vi "SensorSerialReceiver.vi"(8 "Notifier Error In":errorcluster, 9 "Notifier":refnum<notifier>, 10 "Queue":refnum<queue>, 11 "COM Port":refnum<visa-resource-name>="COM6") -> (0 "Notifier Error Out":errorcluster, 3 "Done":bool=TRUE)   [LabVIEW 2013]
uses:
  <vilib>/Instr/_visa.llb/VISA Configure Serial Port (Instr).vi
panel:
  in  "baud rate":u32=115200
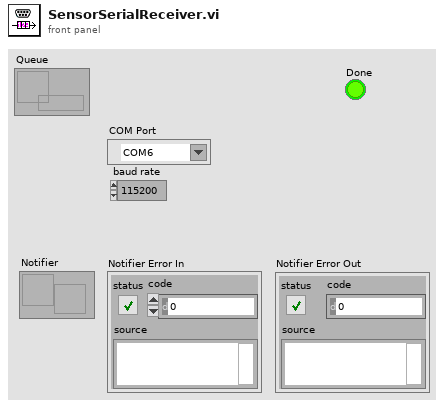
[diagram p1: front panel]
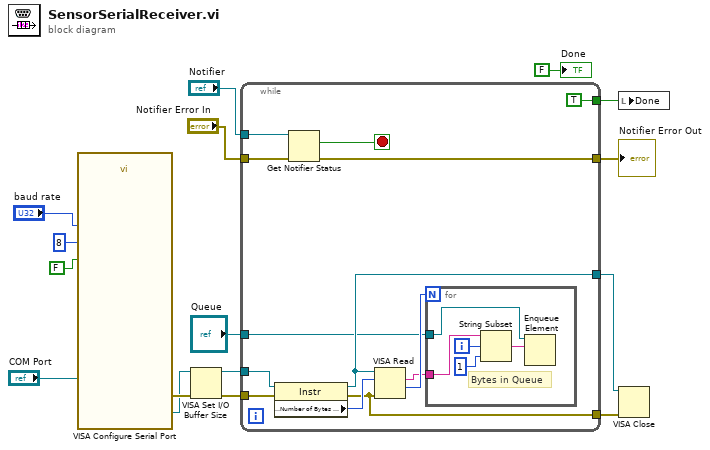
[diagram p0: block diagram]
diagram:
  n1 = call-poly "VISA Configure Serial Port"("VISA resource name"="COM Port", "Enable Termination\nChar (T)"=FALSE ("Enable Termination\nChar (T)"), "baud rate (9600)"="baud rate", "data bits (8)"=u16 8) -> ("VISA resource name out"=w9:refnum<visa-resource-name>, "error out"=w10:errorcluster)  [unwired: 10 in]
  n2 = VISA Set I/O Buffer Size(VISA resource name=w9, error in (no error)=w10) -> (VISA resource name out=w11:refnum<visa-resource-name>, error out=w12:errorcluster)  [unwired: 2 in]
  n3 = while {
    tunnel: w11 -> [w29]
    tunnel: w12 -> [w28]
    tunnel: [w26] -> w14
    tunnel: [w25] -> w15
    tunnel: "Queue" -> [w18]
    tunnel: "Notifier" -> [w22]
    tunnel: "Notifier Error In" -> [w20]
    tunnel: [w19] -> w3
    tunnel: [TRUE] -> w2
    stop <- w21 stop-if-true
    n4 = property class="Instr"(reference=w29, error in=w28) -> (reference out=w26:refnum<visa-resource-name>, error out=w25:errorcluster, "Serial Settings:Number of Bytes at Serial Port"=w27:u32)
    n5 = Get Notifier Status(notifier=w22, error in (no error)=w20) -> (current notification=w21:bool, error out=w19:errorcluster)  [unwired: 3 out]
    n6 = VISA Read(VISA resource name=w26, byte count=w27, error in (no error)=w25) -> (read buffer=w23:string, return count=w24:u32)  [unwired: 2 out]
    n7 = for {
      N: w24 -> [_]
      tunnel: w23 -> [w34]
      tunnel: w18 -> [w31]
      i -> [w33]
      # "Bytes in Queue"
      n8 = String Subset(string=w34, offset (0)=w33, length (rest)=1 ("length (rest)")) -> (substring=w30:string)
      n9 = Enqueue Element(queue=w31, element=w30) -> ()  [unwired: 2 in, 3 out]
    }
  }
  "Notifier Error Out" <- w3
  n10 = local write "Done"(w2) -> ()
  n11 = VISA Close(VISA resource name=w14, error in (no error)=w15) -> ()  [unwired: 1 out]
  "Done" <- FALSE ("Done")
